vi "Unflatten Load & Unload.vi"(8 "Error In":errorcluster, 11 "String":string) -> (0 "Error Out":errorcluster, 3 "Load & Unload.lvclass":refnum<class "Load & Unload.lvclass">)   [LabVIEW 2020, in "lv_icon.lvlib"]
uses:
  resource/plugins/lv_icon.lvlib
  Classes/Load_Unload/Load & Unload.lvclass
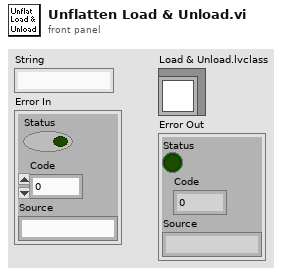
[diagram p1: front panel]
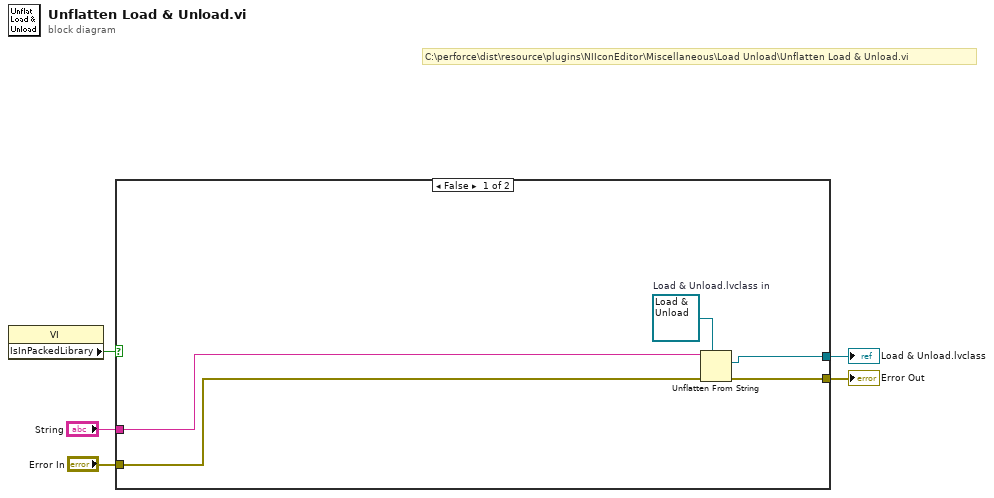
[diagram p0: block diagram]
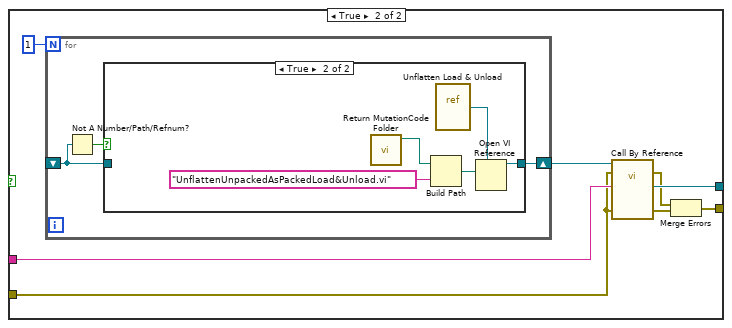
[diagram p2: hidden frame]
diagram:
  # "C:\\perforce\\dist\\resource\\plugins\\NIIconEditor\\Miscellaneous\\Load Unload\\Unflatten Load & Unload.vi"
  n1 = property class="VI"() -> ("IsInPackedLibrary"=w1:bool)  [unwired: 2 in, 2 out]
  n2 = case shown="False" w1 {
    tunnel: "String" -> [w7 w16]
    tunnel: [w8 w15] -> w4
    tunnel: [w9 w13] -> w3
    tunnel: "Error In" -> [w6 w11]
    frame False {
      w10 = refnum<class "Load & Unload.lvclass"> refnum  # Load & Unload.lvclass in
      n3 = Unflatten From String(type=w10, binary string=w7, error in (no error)=w6) -> (value=w8:refnum<class "Load & Unload.lvclass">, error out=w9:errorcluster)  [unwired: 2 in, 1 out]
    }
    frame True {
      n4 = for {
        N: 1 -> [_]
        shift-right: [w19] -> w17
        shift-left: _ -> [w20]
        n5 = Not A Number/Path/Refnum?(number/path/refnum=w20) -> (NaN/Path/Refnum?=w21:bool)
        n6 = case shown="True" w21 {
          tunnel: [w22 w25] -> w19
          tunnel: w20 -> [w22 _]
          frame False {
          }
          frame True {
            n7 = call "Return MutationCode Folder.vi"() -> ("Base Path Mutation Code"=w24:path)  [unwired: 11 in]
            n8 = Build Path(base path=w24, name or relative path="UnflattenUnpackedAsPackedLoad&Unload.vi") -> (appended path=w26:path)
            n9 = vi-ref "Unflatten Load & Unload.vi"() -> (w23:refnum<vi>)
            n10 = Open VI Reference(type specifier VI Refnum (for type only)=w23, vi path=w26) -> (vi reference=w25:refnum<vi>)  [unwired: 4 in, 1 out]
          }
        }
      }
      n11 = call-by-ref "?"(reference=w17, error in=w11, "Error In"=w11, "String"=w16) -> (error out=w12:errorcluster, "Error Out"=w14:errorcluster, "Load & Unload.lvclass"=w15:refnum<class "Load & Unload.lvclass">)  [unwired: 8 in, 1 out]
      n12 = Merge Errors(w12, w14) -> (w13:errorcluster)
    }
  }
  "Load & Unload.lvclass" <- w4
  "Error Out" <- w3
